vi "ReadSourcesNode.vi"(8 "Error In":errorcluster, 11 "Keithley2602 Node In":refnum<k20>) -> (0 "Error Out":errorcluster, 2 "Sources Configuration":T1[](array[typedef]), 3 "Keithley2602 Node Out":refnum<k20>)   [LabVIEW 2013]
uses:
  SourceConfiguration.ctl
  SourceFunction.ctl
  <vilib>/xml/NI_XML.lvlib
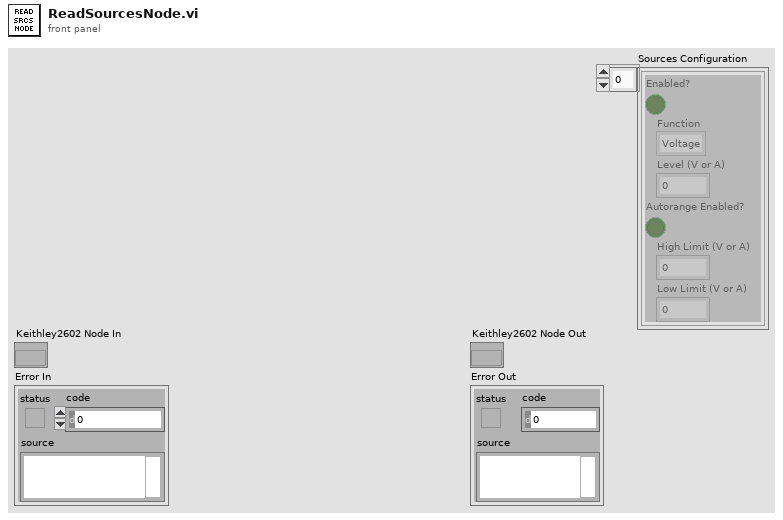
[diagram p1: front panel]
types:
  T1 = typedef "SourceConfiguration.ctl" = cluster{"Enabled?":bool, "Function":T2, "Level (V or A)":dbl, "Autorange Enabled?":bool, "High Limit (V or A)":dbl, "Low Limit (V or A)":dbl}
  T2 = typedef "SourceFunction.ctl" = enum16{"Voltage", "Current"}
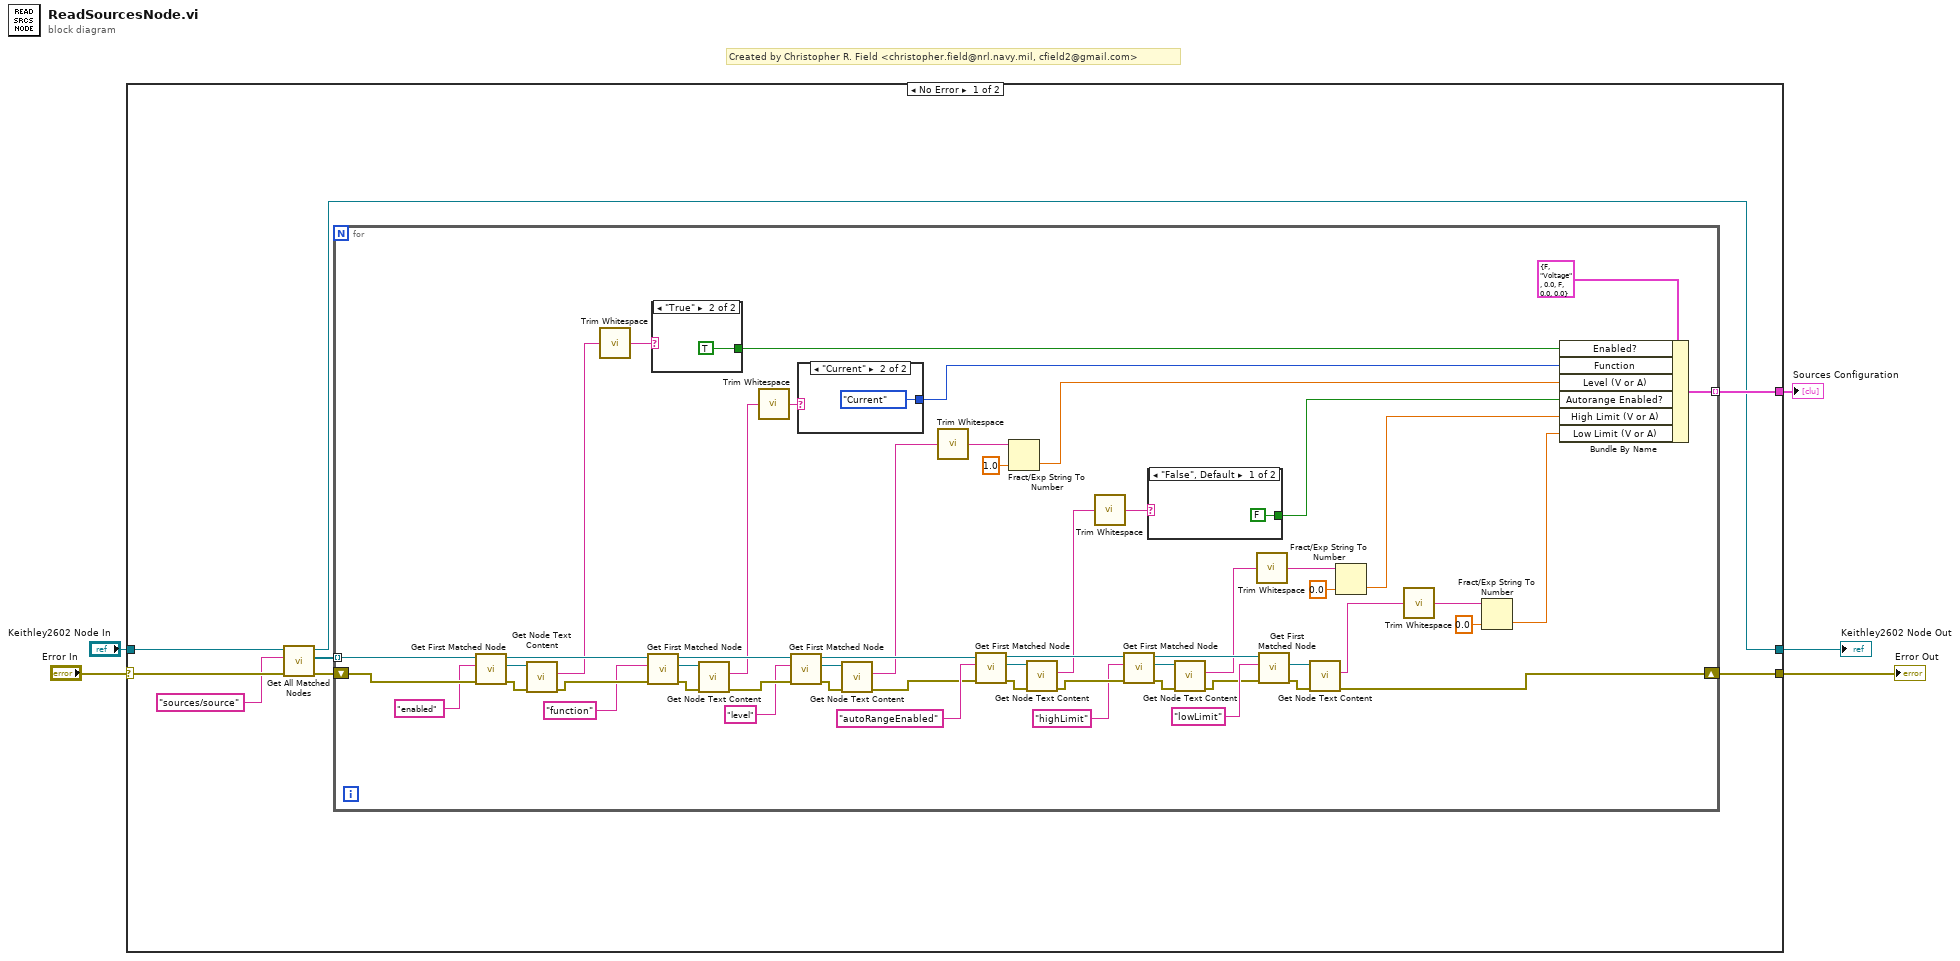
[diagram p0: block diagram]
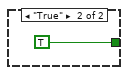
[diagram p2: hidden frame]
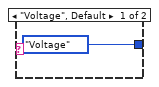
[diagram p3: hidden frame]
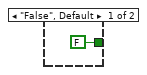
[diagram p4: hidden frame]
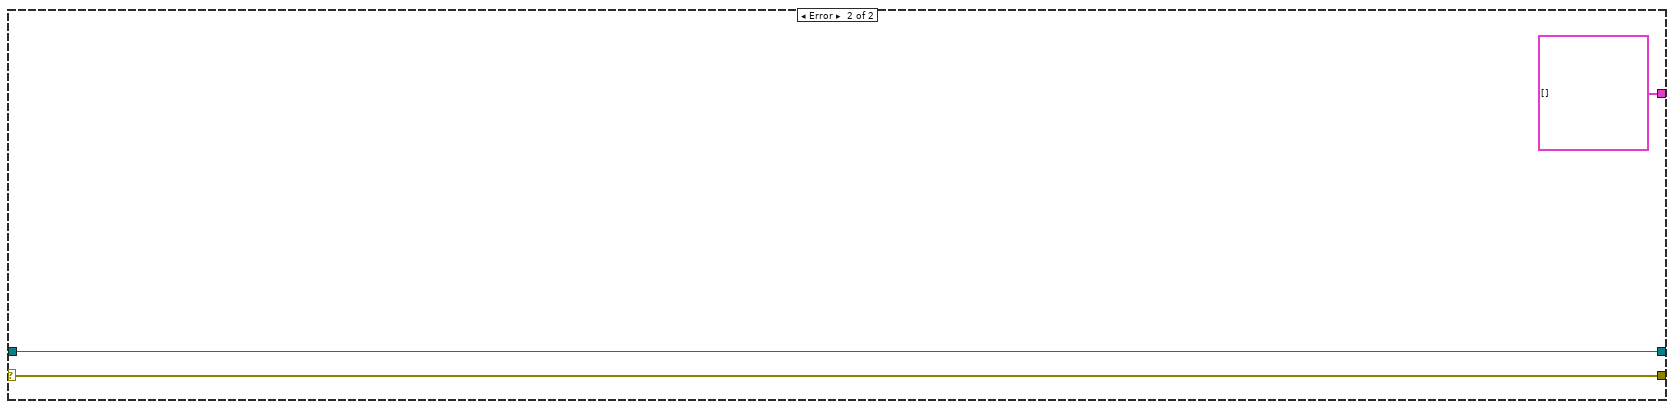
[diagram p5: hidden frame]
diagram:
  # "Created by Christopher R. Field <christopher.field@nrl.navy.mil, cfield2@gmail.com>"
  n1 = case shown="No Error" "Error In" {
    selector: "Error In" -> [w12 w75]
    tunnel: "Keithley2602 Node In" -> [w13 w76]
    tunnel: [w6 w76] -> w3
    tunnel: [w7 w75] -> w2
    tunnel: [w8 T1[] []] -> w1
    frame No Error {
      n2 = call <vilib>:"Get All Matched Nodes.vi"("error in (no error)"=w12, "XPath expression"="sources/source", "node in"=w13) -> ("error out"=w9:errorcluster, "node result array"=w10:refnum<k20>[], "node out"=w6:refnum<k20>)  [unwired: 6 in]
      n3 = for {
        tunnel: w10 -> [w65] mode=indexing
        shift-right: [w29] -> w7
        shift-left: w9 -> [w64]
        tunnel: [w66] -> w8 mode=indexing
        n4 = call <vilib>:"Get First Matched Node.vi"("error in (no error)"=w64, "XPath expression"="enabled", "node in"=w65) -> ("error out"=w61:errorcluster, "node result"=w62:refnum<k20>, "node out"=w57:refnum<k20>)  [unwired: 6 in]
        n5 = call <vilib>:"Get Node Text Content.vi"("error in (no error)"=w61, "node in"=w62) -> ("error out"=w56:errorcluster, "node text"=w24:string)  [unwired: 7 in, 1 out]
        n6 = call <vilib>:"Trim Whitespace.vi"("string"=w24) -> ("trimmed string"=w25:string)  [unwired: 1 in]
        n7 = call <vilib>:"Get First Matched Node.vi"("error in (no error)"=w56, "XPath expression"="function", "node in"=w57) -> ("error out"=w58:errorcluster, "node result"=w59:refnum<k20>, "node out"=w51:refnum<k20>)  [unwired: 6 in]
        n8 = case shown="\"True\"" w25 {
          tunnel: [FALSE TRUE] -> w60
          frame "False", Default {
          }
          frame "True" {
          }
        }
        n9 = call <vilib>:"Get Node Text Content.vi"("error in (no error)"=w58, "node in"=w59) -> ("error out"=w50:errorcluster, "node text"=w22:string)  [unwired: 7 in, 1 out]
        n10 = call <vilib>:"Trim Whitespace.vi"("string"=w22) -> ("trimmed string"=w23:string)  [unwired: 1 in]
        n11 = call <vilib>:"Get First Matched Node.vi"("error in (no error)"=w50, "XPath expression"="level", "node in"=w51) -> ("error out"=w52:errorcluster, "node result"=w53:refnum<k20>, "node out"=w44:refnum<k20>)  [unwired: 6 in]
        n12 = case shown="\"Current\"" w23 {
          tunnel: [SourceFunction."Voltage" ("Function") SourceFunction."Current" ("Function")] -> w54
          frame "Voltage", Default {
          }
          frame "Current" {
          }
        }
        n13 = call <vilib>:"Get Node Text Content.vi"("error in (no error)"=w52, "node in"=w53) -> ("error out"=w43:errorcluster, "node text"=w20:string)  [unwired: 7 in, 1 out]
        n14 = call <vilib>:"Trim Whitespace.vi"("string"=w20) -> ("trimmed string"=w21:string)  [unwired: 1 in]
        n15 = call <vilib>:"Get First Matched Node.vi"("error in (no error)"=w43, "XPath expression"="autoRangeEnabled", "node in"=w44) -> ("error out"=w46:errorcluster, "node result"=w47:refnum<k20>, "node out"=w37:refnum<k20>)  [unwired: 6 in]
        n16 = Fract/Exp String To Number(string=w21, default (0 dbl)=1.0 ("default (0 DBL)")) -> (number=w48:dbl)  [unwired: 2 in, 1 out]
        n17 = call <vilib>:"Get Node Text Content.vi"("error in (no error)"=w46, "node in"=w47) -> ("error out"=w36:errorcluster, "node text"=w18:string)  [unwired: 7 in, 1 out]
        n18 = call <vilib>:"Trim Whitespace.vi"("string"=w18) -> ("trimmed string"=w19:string)  [unwired: 1 in]
        n19 = call <vilib>:"Get First Matched Node.vi"("error in (no error)"=w36, "XPath expression"="highLimit", "node in"=w37) -> ("error out"=w40:errorcluster, "node result"=w41:refnum<k20>, "node out"=w33:refnum<k20>)  [unwired: 6 in]
        n20 = case shown="\"False\", Default" w19 {
          tunnel: [FALSE TRUE] -> w42
          frame "False", Default {
          }
          frame "True" {
          }
        }
        n21 = call <vilib>:"Get Node Text Content.vi"("error in (no error)"=w40, "node in"=w41) -> ("error out"=w31:errorcluster, "node text"=w16:string)  [unwired: 7 in, 1 out]
        n22 = call <vilib>:"Trim Whitespace.vi"("string"=w16) -> ("trimmed string"=w17:string)  [unwired: 1 in]
        n23 = call <vilib>:"Get First Matched Node.vi"("error in (no error)"=w31, "XPath expression"="lowLimit", "node in"=w33) -> ("error out"=w38:errorcluster, "node result"=w39:refnum<k20>)  [unwired: 6 in, 1 out]
        n24 = call <vilib>:"Get Node Text Content.vi"("error in (no error)"=w38, "node in"=w39) -> ("error out"=w29:errorcluster, "node text"=w14:string)  [unwired: 7 in, 1 out]
        n25 = Fract/Exp String To Number(string=w17, default (0 dbl)=0.0 ("default (0 DBL)")) -> (number=w34:dbl)  [unwired: 2 in, 1 out]
        n26 = call <vilib>:"Trim Whitespace.vi"("string"=w14) -> ("trimmed string"=w15:string)  [unwired: 1 in]
        n27 = Fract/Exp String To Number(string=w15, default (0 dbl)=0.0 ("default (0 DBL)")) -> (number=w30:dbl)  [unwired: 2 in, 1 out]
        n28 = Bundle By Name(cluster=T1 {"Enabled?"=FALSE, "Function"=enum."Voltage", "Level (V or A)"=0.0, "Autorange Enabled?"=FALSE, "High Limit (V or A)"=0.0, "Low Limit (V or A)"=0.0} ("Source Configuration"), "Enabled?"=w60, "Function"=w54, "Level (V or A)"=w48, "Autorange Enabled?"=w42, "High Limit (V or A)"=w34, "Low Limit (V or A)"=w30) -> (w66:T1)
      }
    }
    frame Error {
    }
  }
  "Keithley2602 Node Out" <- w3
  "Error Out" <- w2
  "Sources Configuration" <- w1
